vi "Load Repos from file.vi"(8 "error in":errorcluster) -> (0 "error out":errorcluster, 3 "Repos":refnum<class "Repo.lvclass">[](array[class]))   [LabVIEW 2020, in "WSsupport.lvlib"]
uses:
  WSsupport.lvlib
  Packages/Repo_class/Repo.lvclass
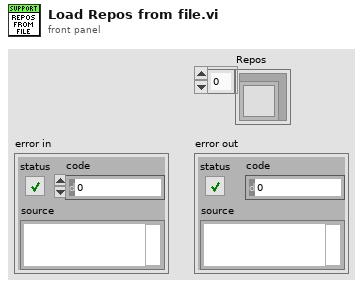
[diagram p1: front panel]
types:
  T1 = enum16{"open", "replace", "create", "open or create", "replace or create", "replace or create with confirmation"}
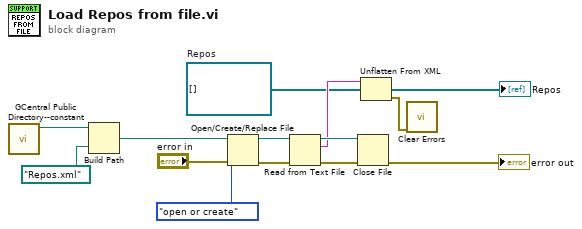
[diagram p0: block diagram]
diagram:
  w5 = refnum<class "Repo.lvclass">[] []  # Repos
  n1 = call "GCentral Public Directory--constant.vi"() -> ("GCentral Public Dir"=w14:path)  [unwired: 11 in]
  n2 = Build Path(base path=w14, name or relative path=path "Repos.xml") -> (appended path=w12:path)
  n3 = Open/Create/Replace File(file path (use dialog)=w12, error in="error in", operation (0:open)=T1."open or create") -> (refnum out=w10:refnum<file>, error out=w9:errorcluster)  [unwired: 3 in, 1 out]
  n4 = Read from Text File(file (use dialog)=w10, error in=w9) -> (refnum out=w8:refnum<file>, text=w6:string, error out=w7:errorcluster)  [unwired: 2 in, 1 out]
  n5 = Close File(refnum=w8, error in=w7) -> (error out=→"error out":errorcluster)  [unwired: 1 out]
  n6 = Unflatten From XML(xml string=w6, type=w5) -> (value=→"Repos":refnum<class "Repo.lvclass">[], error out=w4:errorcluster)  [unwired: 1 in]
  n7 = call <vilib>:"Clear Errors.vi"("error in (no error)"=w4) -> ()  [unwired: 5 in, 2 out]
